vi "FLASH.vi"   [LabVIEW 2023]
uses:
  Application/Application.lvclass
  C:/Program Files/National Instruments/LabVIEW 2023/vi.lib/ActorFramework/Actor/Actor.lvclass
  <vilib>/ActorFramework/Actor/Actor.lvclass
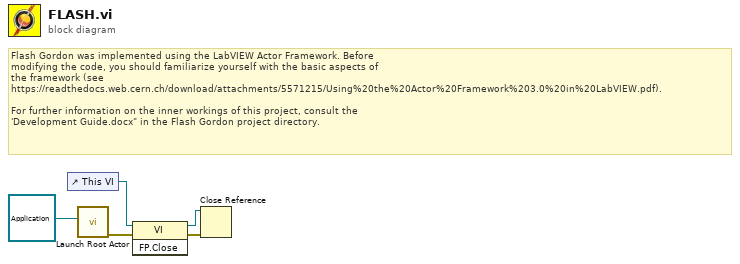
[diagram p0: block diagram]
diagram:
  # "Flash Gordon was implemented using the LabVIEW Actor Framework. Before\nmodifying the code, you should familiarize yourself with the basic aspects of \nthe framework (see\nhttps://readthedocs.web.cern.ch/download/attachments/5571215/Using%20the%20Actor%20Framework%203.0%20in%20LabVIEW.pdf).\n\nFor further information on the inner workings of this project, consult the \n'Development Guide.docx\" in the Flash Gordon project directory."
  n1 = control-ref of="This VI"() -> (w2:refnum<vi>)
  n2 = call <vilib>:"Launch Root Actor.vi"("Actor"=refnum<class "Application.lvclass"> refnum ("Application.lvlib:Application.lvclass")) -> ("error out"=w1:errorcluster)  [unwired: 9 in, 1 out]
  n3 = invoke class="VI" method="FP.Close"(reference=w2, error in=w1) -> (reference out=w4:refnum<vi>, error out=w3:errorcluster)  [unwired: 1 in, 1 out]
  n4 = Close Reference(reference=w4, error in (no error)=w3) -> ()  [unwired: 1 out]
